vi "Joystick Deadbander.vi"(6 "Invert (TF)":bool, 8 "y":dbl, 11 "x":dbl) -> (0 "y edited":dbl, 3 "X edited":dbl)   [LabVIEW 2012]
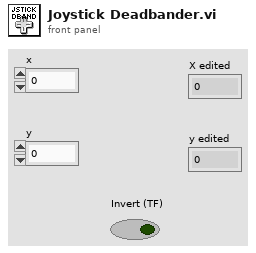
[diagram p1: front panel]
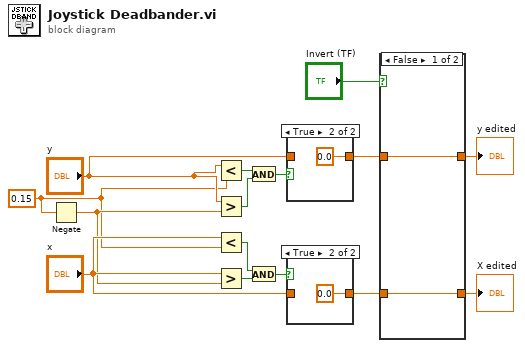
[diagram p0: block diagram]
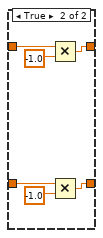
[diagram p2: hidden frame]
diagram:
  w1 = 0.15 ("y")
  n1 = Negate(x=w1) -> (-x=w5:dbl)
  n2 = Less?(x="y", y=w1) -> (x < y?=w3:bool)
  n3 = Greater?(x="y", y=w5) -> (0:w4:bool)
  n4 = Less?(x="x", y=w1) -> (x < y?=w7:bool)
  n5 = Greater?(x="x", y=w5) -> (0:w6:bool)
  n6 = And(x=w3, y=w4) -> (x .and. y?=w13:bool)
  n7 = And(x=w7, y=w6) -> (x .and. y?=w15:bool)
  n8 = case shown="True" w13 {
    tunnel: "y" -> [w16 _]
    tunnel: [w16 0.0] -> w10
    frame False {
    }
    frame True {
    }
  }
  n9 = case shown="True" w15 {
    tunnel: "x" -> [w18 _]
    tunnel: [w18 0.0] -> w11
    frame False {
    }
    frame True {
    }
  }
  n10 = case shown="False" "Invert (TF)" {
    tunnel: w11 -> [w21 w23]
    tunnel: [w21 w22] -> w8
    tunnel: w10 -> [w20 w25]
    tunnel: [w20 w24] -> w9
    frame False {
    }
    frame True {
      n11 = Multiply(x=w25, y=-1.0) -> (x*y=w24:dbl)
      n12 = Multiply(x=w23, y=-1.0) -> (x*y=w22:dbl)
    }
  }
  "X edited" <- w8
  "y edited" <- w9
